vi "Connect.vi"(8 "error in":errorcluster, 11 "Newport in":refnum<class "Newport.lvclass">) -> (0 "error out":errorcluster, 3 "Newport out":refnum<class "Newport.lvclass">)   [LabVIEW 2018, in "Newport.lvlib" / "Newport.lvclass"]
uses:
  Newport.lvclass
  C:/Projects/LabVIEW/In-Progress/Chetan Malpure/Axis/Parent/Axis.lvclass
  Parent/Axis.lvclass/Axis.ctl
  Newport.XPS.CommandInterface
  Parent/Axis.lvclass
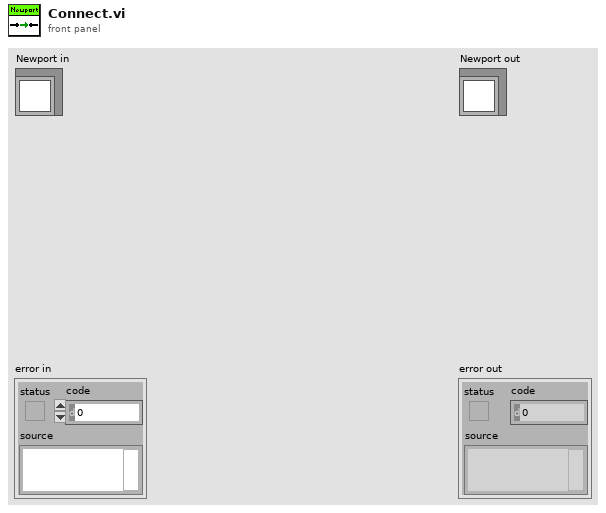
[diagram p1: front panel]
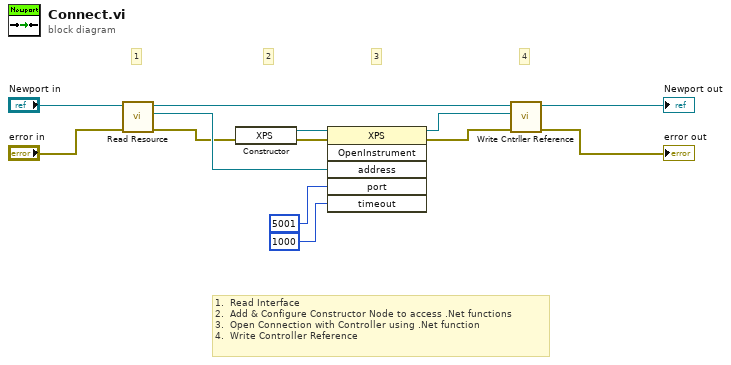
[diagram p0: block diagram]
diagram:
  # "1.  Read Interface\n2.  Add & Configure Constructor Node to access .Net functions\n3.  Open Connection with Controller using .Net function\n4.  Write Controller Reference"
  # "4"
  # "3"
  # "2"
  # "1"
  n1 = call "Read Resource.vi"("error in"="error in", "Axis in"="Newport in") -> ("error out"=w9:errorcluster, "Resource"=w12:refnum<visa-resource-name>, "Axis out"=w3:refnum<class "Newport.lvclass">)  [unwired: 7 in]
  n2 = constructor class="XPS"(error in=w9) -> (reference out=w11:refnum<k24>, error out=w10:errorcluster)  [unwired: 2 in, 1 out]
  n3 = invoke class="XPS" method="OpenInstrument"(reference=w11, error in=w10, "address"=w12, "port"=5001, "timeout"=1000) -> (reference out=w5:refnum<k24>, error out=w4:errorcluster)  [unwired: 1 in, 4 out]
  n4 = call-dynamic "Write Cntrller Reference.vi"("error in (no error)"=w4, "Cntrller Reference"=w5, "Newport in"=w3) -> ("error out"=→"error out":errorcluster, "Newport out"=→"Newport out":refnum<class "Newport.lvclass">)  [unwired: 7 in]
